vi "Register gRPC Methods.vi"(8 "error in (no error)":errorcluster, 11 "Template Server in":refnum<class "NW and PSD_server.lvclass">) -> (0 "error out":errorcluster, 3 "Template Server out":refnum<class "NW and PSD_server.lvclass">)   [LabVIEW 2019, in "NW and PSD_server.lvlib" / "NW and PSD_server.lvclass"]
uses:
  NW and PSD_server.lvclass
  typeDefs/Server Internal UEs.ctl
  typeDefs/Server Internal Message.ctl
  typeDefs/Server gRPC UEs.ctl
  <vilib>/gRPC/LabVIEW gRPC Library/Server API/typeDefs/gRPCId Cluster.ctl
  <vilib>/gRPC/LabVIEW gRPC Library/Server API/typeDefs/grpcId.ctl
  NW and PSD_server.lvclass/NW and PSD_server.ctl
  <vilib>/gRPC/LabVIEW gRPC Library/gprc-lvsupport-release.lvlib
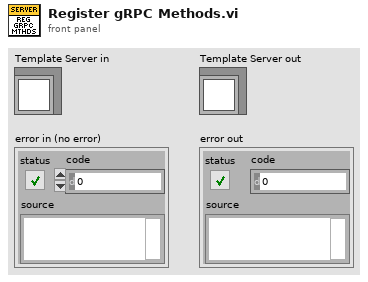
[diagram p1: front panel]
types:
  T1 = typedef "NW and PSD_server.lvlib/NW and PSD_server.lvclass/Server gRPC UEs.ctl" = cluster{"example_SignalGeneratorService_ApplySignalParameters gRPC UE":refnum<user-event>, "example_SignalGeneratorService_ApplyNoiseParameters gRPC UE":refnum<user-event>, "example_SignalGeneratorService_GenerateSignal gRPC UE":refnum<user-event>, "example_SignalGeneratorService_GetAnalyzedParameters gRPC UE":refnum<user-event>}
  T2 = typedef "NW and PSD_server.lvlib/NW and PSD_server.lvclass/Server Internal UEs.ctl" = cluster{"example_SignalGeneratorService_ApplySignalParameters Internal UE":refnum<user-event>, "example_SignalGeneratorService_ApplyNoiseParameters Internal UE":refnum<user-event>, "example_SignalGeneratorService_GenerateSignal Internal UE":refnum<user-event>, "example_SignalGeneratorService_GetAnalyzedParameters Internal UE":refnum<user-event>}
  T3 = typedef "gprc-lvsupport-release.lvlib/grpcId.ctl" = u64
  T4 = typedef "NW and PSD_server.lvlib/NW and PSD_server.lvclass/Server Internal Message UE.ctl" = refnum<user-event>
  T5 = typedef "gprc-lvsupport-release.lvlib/gRPCId Cluster UE.ctl" = refnum<user-event>
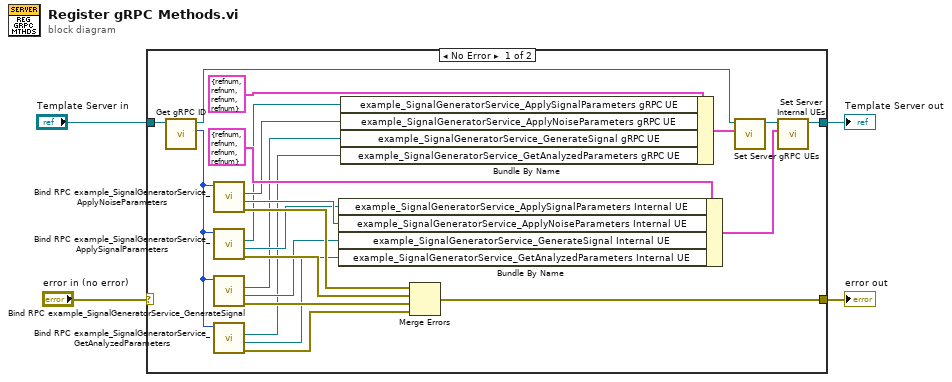
[diagram p0: block diagram]
diagram:
  n1 = case shown="No Error" "error in (no error)" {
    selector: "error in (no error)" -> [_ w27]
    tunnel: "Template Server in" -> [w25 w28]
    tunnel: [w24 w27] -> w3
    tunnel: [w23 w28] -> w2
    frame No Error {
      n2 = call "Get gRPC ID.vi"("OOP Server in"=w25) -> ("gRPC ID"=w17:T3, "OOP Server out"=w26:refnum<class "NW and PSD_server.lvclass">)  [unwired: 9 in]
      n3 = call "Bind RPC example_SignalGeneratorService_ApplyNoiseParameters.vi"("gRPCid server in"=w17) -> ("error out"=w16:errorcluster, "example_SignalGeneratorService_ApplyNoiseParameters Internal UE"=w14:T4, "example_SignalGeneratorService_ApplyNoiseParameters gRPC UE"=w15:T5)  [unwired: 7 in, 1 out]
      n4 = call "Bind RPC example_SignalGeneratorService_ApplySignalParameters.vi"("gRPCid server in"=w17) -> ("error out"=w13:errorcluster, "example_SignalGeneratorService_ApplySignalParameters Internal UE"=w11:T4, "example_SignalGeneratorService_ApplySignalParameters gRPC UE"=w12:T5)  [unwired: 7 in, 1 out]
      n5 = call "Bind RPC example_SignalGeneratorService_GenerateSignal.vi"("gRPCid server in"=w17) -> ("error out"=w10:errorcluster, "example_SignalGeneratorService_GenerateSignal Internal UE"=w8:T4, "example_SignalGeneratorService_GenerateSignal gRPC UE"=w9:T5)  [unwired: 7 in, 1 out]
      n6 = call "Bind RPC example_SignalGeneratorService_GetAnalyzedParameters.vi"("gRPCid server in"=w17) -> ("error out"=w7:errorcluster, "example_SignalGeneratorService_GetAnalyzedParameters Internal UE"=w5:T4, "example_SignalGeneratorService_GetAnalyzedParameters gRPC UE"=w6:T5)  [unwired: 7 in, 1 out]
      n7 = Bundle By Name ("Bundle Internal UEs")(cluster=T2 {"example_SignalGeneratorService_ApplySignalParameters Internal UE"=refnum, "example_SignalGeneratorService_ApplyNoiseParameters Internal UE"=refnum, "example_SignalGeneratorService_GenerateSignal Internal UE"=refnum, "example_SignalGeneratorService_GetAnalyzedParameters Internal UE"=refnum} ("Server Internal UEs"), "example_SignalGeneratorService_ApplySignalParameters Internal UE"=w11, "example_SignalGeneratorService_ApplyNoiseParameters Internal UE"=w14, "example_SignalGeneratorService_GenerateSignal Internal UE"=w8, "example_SignalGeneratorService_GetAnalyzedParameters Internal UE"=w5) -> (w22:T2)
      n8 = Bundle By Name ("Bundle gRPC UEs")(cluster=T1 {"example_SignalGeneratorService_ApplySignalParameters gRPC UE"=refnum, "example_SignalGeneratorService_ApplyNoiseParameters gRPC UE"=refnum, "example_SignalGeneratorService_GenerateSignal gRPC UE"=refnum, "example_SignalGeneratorService_GetAnalyzedParameters gRPC UE"=refnum} ("gRPC Server Method Events"), "example_SignalGeneratorService_ApplySignalParameters gRPC UE"=w12, "example_SignalGeneratorService_ApplyNoiseParameters gRPC UE"=w15, "example_SignalGeneratorService_GenerateSignal gRPC UE"=w9, "example_SignalGeneratorService_GetAnalyzedParameters gRPC UE"=w6) -> (w19:T1)
      n9 = Merge Errors(w16, w13, w10, w7) -> (w24:errorcluster)
      n10 = call "Set Server gRPC UEs.vi"("Server RPC Methods"=w19, "OOP Server in"=w26) -> ("OOP Server out"=w20:refnum<class "NW and PSD_server.lvclass">)  [unwired: 9 in]
      n11 = call "Set Server Internal UEs.vi"("Server Internal UEs"=w22, "OOP Server in"=w20) -> ("OOP Server out"=w23:refnum<class "NW and PSD_server.lvclass">)  [unwired: 9 in]
    }
    frame Error {
    }
  }
  "error out" <- w3
  "Template Server out" <- w2
